vi "Create Base Queue.vi"(9 "Queue jettl":refnum<class "Queue.lvclass">, 10 "Alias":string) -> (0 "error out":errorcluster)   [LabVIEW 2021, in "jettl.lvlib" / "Base Queue jettl.lvlib"]
uses:
  Base Queue jettl.lvlib
  Base Queue jettl/Base Queue jettl.lvclass
  Queue/Queue.lvclass
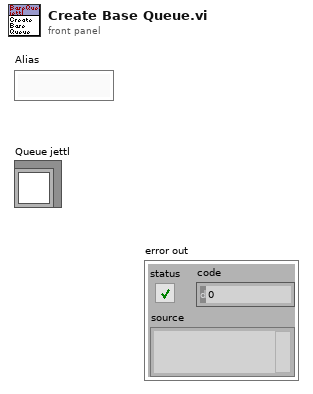
[diagram p1: front panel]
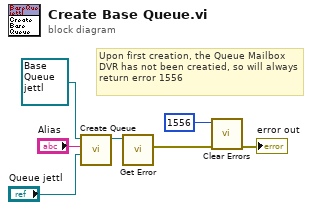
[diagram p0: block diagram]
diagram:
  # "Upon first creation, the Queue Mailbox DVR has not been creatied, so will always return error 1556"
  n1 = call-dynamic "Create Queue.vi"("Queue jettl"="Queue jettl", "Alias"="Alias", "Base Queue jettl in"=refnum<class "Base Queue jettl.lvclass"> refnum ("jettl Queue Actor.lvlib:jettl Queue Actor.lvclass")) -> ("Base Queue jettl out"=w6:refnum<class "Base Queue jettl.lvclass">)  [unwired: 8 in]
  n2 = call-dynamic "Get Error.vi"("Base Queue jettl in"=w6) -> ("Error"=w2:errorcluster)  [unwired: 10 in]
  n3 = call <vilib>:"Clear Errors.vi"("error in (no error)"=w2, "specific error code to clear (0: all)"=1556) -> ("error out"=→"error out":errorcluster)  [unwired: 4 in, 1 out]
